vi "Undersample_Core.vi"(0 "U/S Location":string(combo)="VCO", 5 "U/S Frequency":i32=2400, 7 "Unit Info":string="Unit1", 9 "Core PLL Instance":string(combo)="Core0", 11 "error in (no error)":errorcluster) -> (4 "Total RMS Jitter":string, 6 "Cycle-Cycle Jitter":string, 15 "error out":errorcluster)   [LabVIEW 2011]
doc: "This VI undersamples a selected signal from a selected Core PLL instance at a specified frequency.\n\nInputs:\n1. U/S Location: Part of PLL loop to be undersamles (VCO, PllOut, VCO_Z, Spine, etc).\n2. U/S Frequency: Frequency at which the PLL to be undersampled is running (2400, 2600, etc.)\n3. Unit Info: Information about the unit to attach to undersampling results file.\n4. Core PLL Instance: Instance of the Core PLL to undersample (Core0, Core1, etc.)\n\nOutputs:\n1. Total RMS Jitter: The total RMS Jitter as read from the resultspectrum file.\n2. Cycle-Cycle Jitter: The Cycle-Cycle Jitter as read from the result spectrum file."
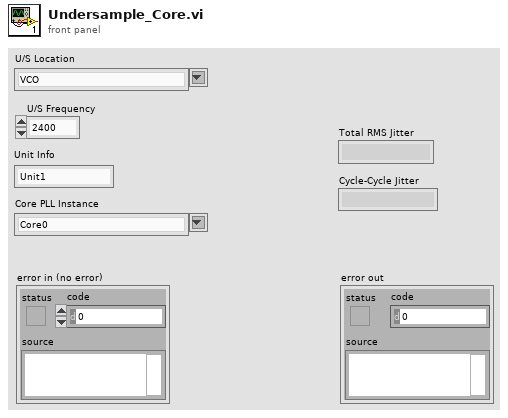
[diagram p1: front panel]
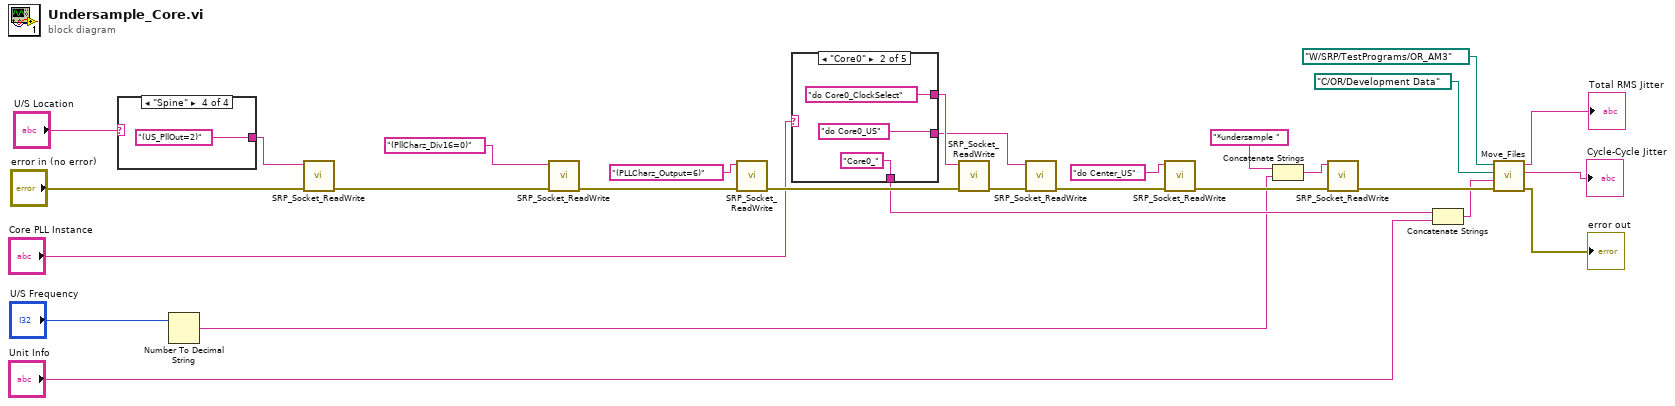
[diagram p0: block diagram]
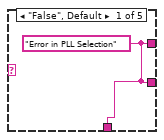
[diagram p2: hidden frame]
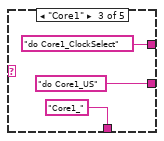
[diagram p3: hidden frame]
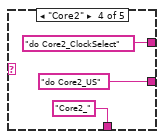
[diagram p4: hidden frame]
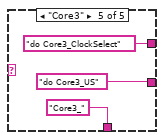
[diagram p5: hidden frame]
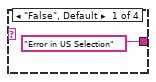
[diagram p6: hidden frame]
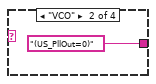
[diagram p7: hidden frame]
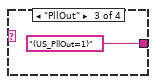
[diagram p8: hidden frame]
diagram:
  n1 = case shown="\"Spine\"" "U/S Location" {
    tunnel: ["Error in US Selection" "(US_PllOut=0)" "(US_PllOut=1)" "(US_PllOut=2)"] -> w5
    frame "False", Default {
    }
    frame "VCO" {
    }
    frame "PllOut" {
    }
    frame "Spine" {
    }
  }
  n2 = Number To Decimal String(number="U/S Frequency") -> (decimal integer string=w3:string)  [unwired: 1 in]
  n3 = call "SRP_Socket_ReadWrite.vi"("error in (no error)"="error in (no error)", "Data In"=w5) -> ("error out"=w25:errorcluster)  [unwired: 7 in, 1 out]
  n4 = call "SRP_Socket_ReadWrite.vi"("error in (no error)"=w25, "Data In"="(PllCharz_Div16=0)") -> ("error out"=w24:errorcluster)  [unwired: 7 in, 1 out]
  n5 = call "SRP_Socket_ReadWrite.vi"("error in (no error)"=w24, "Data In"="(PLLCharz_Output=6)") -> ("error out"=w23:errorcluster)  [unwired: 7 in, 1 out]
  n6 = case shown="\"Core0\"" "Core PLL Instance" {
    tunnel: [w33 "do Core0_ClockSelect" "do Core1_ClockSelect" "do Core2_ClockSelect" "do Core3_ClockSelect"] -> w9
    tunnel: [w33 "do Core0_US" "do Core1_US" "do Core2_US" "do Core3_US"] -> w8
    tunnel: [w33 "Core0_" "Core1_" "Core2_" "Core3_"] -> w14
    frame "False", Default {
      w33 = "Error in PLL Selection"
    }
    frame "Core0" {
    }
    frame "Core1" {
    }
    frame "Core2" {
    }
    frame "Core3" {
    }
  }
  n7 = call "SRP_Socket_ReadWrite.vi"("error in (no error)"=w23, "Data In"=w9) -> ("error out"=w20:errorcluster)  [unwired: 7 in, 1 out]
  n8 = call "SRP_Socket_ReadWrite.vi"("error in (no error)"=w20, "Data In"=w8) -> ("error out"=w22:errorcluster)  [unwired: 7 in, 1 out]
  n9 = call "SRP_Socket_ReadWrite.vi"("error in (no error)"=w22, "Data In"="do Center_US") -> ("error out"=w21:errorcluster)  [unwired: 7 in, 1 out]
  n10 = Concatenate Strings("*undersample ", w3) -> (w11:string)
  n11 = call "SRP_Socket_ReadWrite.vi"("error in (no error)"=w21, "Data In"=w11) -> ("error out"=w17:errorcluster)  [unwired: 7 in, 1 out]
  n12 = Concatenate Strings(w14, "Unit Info") -> (w15:string)
  n13 = call "Move_Files.vi"("error in"=w17, "Unit Information"=w15, "Target Directory to Save U/S Files"=path "C:/OR/Development Data", "Location of U/S Files"=path "W:/SRP/TestPrograms/OR_AM3") -> ("error out"=→"error out":errorcluster, "Cycle-Cycle-Jitter"=→"Cycle-Cycle Jitter":string, "Total RMS Jitter"=→"Total RMS Jitter":string)  [unwired: 5 in]
